vi "Bring UI To Front.vi"(11 "UI Data in":refnum<class "Settings UI.lvclass">) -> (0 "error out":errorcluster, 3 "UI Data out":refnum<class "Settings UI.lvclass">)   [LabVIEW 2020, in "Output Sequencer.lvlib" / "Settings UI.lvclass"]
uses:
  Settings UI.lvclass
  Settings UI.lvclass/Settings UI.ctl
  user32.dll
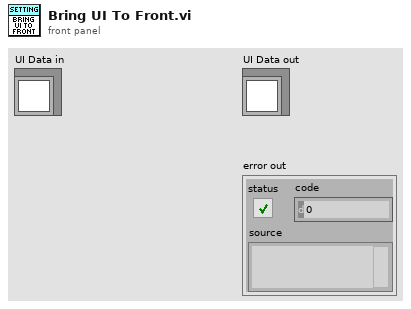
[diagram p1: front panel]
types:
  T1 = enum32{"Invalid", "Standard", "Closed", "Hidden", "Minimized", "Maximized"}
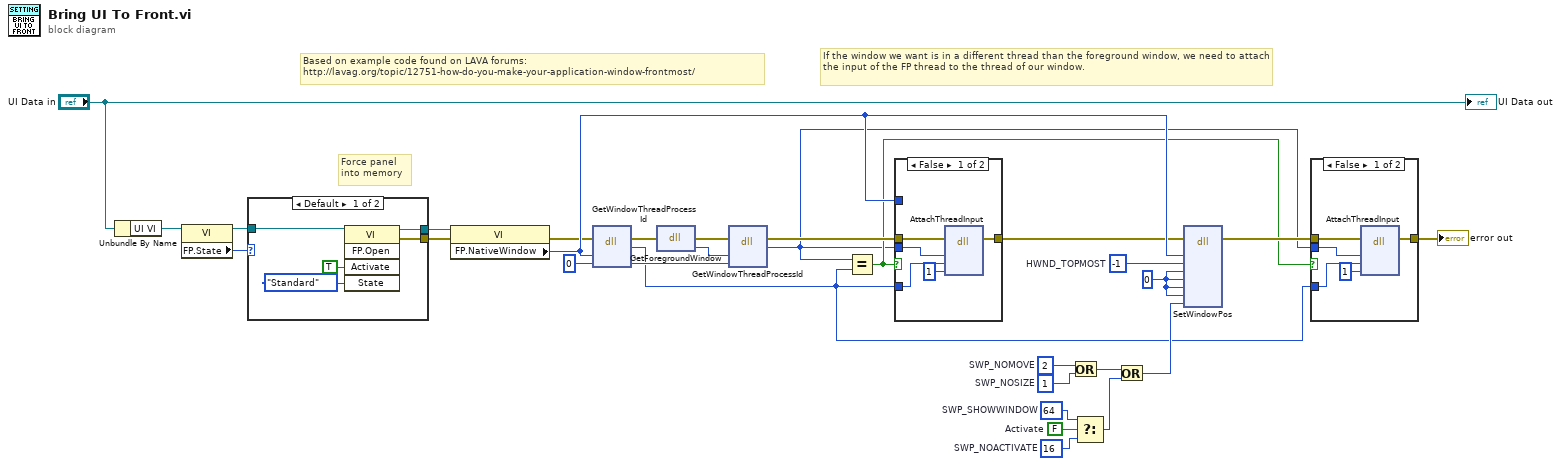
[diagram p0: block diagram]
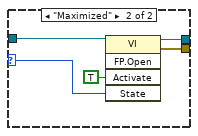
[diagram p2: hidden frame]
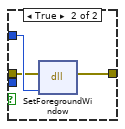
[diagram p4: hidden frame]
diagram:
  w14 = FALSE  # Activate
  w21 = -1  # HWND_TOPMOST
  w13 = u32 16  # SWP_NOACTIVATE
  w12 = u32 64  # SWP_SHOWWINDOW
  w18 = 0 ("lpdwProcessID")
  w26 = u32 2  # SWP_NOMOVE
  w25 = u32 1  # SWP_NOSIZE
  w27 = 0
  # "Force panel\ninto memory"
  # "Based on example code found on LAVA forums:\nhttp://lavag.org/topic/12751-how-do-you-make-your-application-window-frontmost/"
  # "If the window we want is in a different thread than the foreground window, we need to attach the input of the FP thread to the thread of our window."
  n1 = Unbundle By Name("UI Data in") -> ("UI VI"=w2:refnum<vi>)
  n2 = property class="VI"(reference=w2) -> (reference out=w7:refnum<vi>, "FP.State"=w6:T1)  [unwired: 1 in, 1 out]
  n3 = case shown="Default" w6 {
    selector: w6 -> [_ w35]
    tunnel: [w32 w38] -> w29
    tunnel: [w31 w37] -> w28
    tunnel: w7 -> [w30 w36]
    frame Default {
      n4 = invoke class="VI" method="FP.Open"(reference=w30, "Activate"=TRUE ("Activate?"), "State"=T1."Standard") -> (reference out=w31:refnum<vi>, error out=w32:errorcluster)  [unwired: 2 in, 3 out]
    }
    frame "Maximized" {
      n5 = invoke class="VI" method="FP.Open"(reference=w36, "Activate"=TRUE ("Activate?"), "State"=w35) -> (reference out=w37:refnum<vi>, error out=w38:errorcluster)  [unwired: 2 in, 3 out]
    }
  }
  n6 = property class="VI"(reference=w28, error in=w29) -> (error out=w4:errorcluster, "FP.NativeWindow"=w20:u64)  [unwired: 1 out]
  n7 = dll-call lib="user32" fn="GetWindowThreadProcessId" label="Get\nWindow\nThread\nProcess\nId"(error in=w4, "hWnd"=w20, "lpdwProcessID"=w18) -> (error out=w16:errorcluster, w9:i32)  [unwired: 4 in, 1 out]
  n8 = dll-call lib="user32" fn="GetForegroundWindow" label="Get\nForeground\nWindow"(error in=w16) -> (error out=w17:errorcluster, "hWnd"=w19:i32)  [unwired: 2 in, 1 out]
  n9 = dll-call lib="user32" fn="GetWindowThreadProcessId" label="Get\nWindow\nThread\nProcess\nId"(error in=w17, "hWnd"=w19, "lpdwProcessID"=w18) -> (error out=w15:errorcluster, w8:i32)  [unwired: 4 in, 1 out]
  n10 = Equal?(x=w8, y=w9) -> (x = y?=w10:bool)
  n11 = case shown="False" w10 {
    tunnel: w8 -> [w44 _]
    tunnel: w9 -> [w43 _]
    tunnel: w20 -> [_ w47]
    tunnel: w15 -> [w41 w46]
    tunnel: [w40 w45] -> w5
    frame False {
      n12 = dll-call lib="user32" fn="AttachThreadInput" label="Attach\nThread\nInput"(error in=w41, "idAttach"=w44, "idAttachTo"=w43, "fAttach"=1) -> (error out=w40:errorcluster)  [unwired: 6 in, 1 out]
    }
    frame True {
      n13 = dll-call lib="user32" fn="SetForegroundWindow" label="Set\nForeground\nWindow"(error in=w46, "hWnd"=w47) -> (error out=w45:errorcluster)  [unwired: 4 in, 1 out]
    }
  }
  n14 = Or(x=w26, y=w25) -> (x .or. y?=w23:u32)
  n15 = Select(t=w12, s=w14, f=w13) -> (s? t:f=w24:u32)
  n16 = Or(x=w23, y=w24) -> (x .or. y?=w22:u32)
  n17 = dll-call lib="USER32.DLL" fn="SetWindowPos"(error in=w5, "hWnd"=w20, "hWndInsertAfter"=w21, "left"=w27, "top"=w27, "width"=w27, "height"=w27, "fuFlags"=w22) -> (error out=w11:errorcluster)  [unwired: 8 in, 3 out]
  n18 = case shown="False" w10 {
    tunnel: w8 -> [w52 _]
    tunnel: w9 -> [w51 _]
    tunnel: w11 -> [w49 w53]
    tunnel: [w48 w53] -> w3
    frame False {
      n19 = dll-call lib="user32" fn="AttachThreadInput" label="Attach\nThread\nInput"(error in=w49, "idAttach"=w52, "idAttachTo"=w51, "fAttach"=1) -> (error out=w48:errorcluster)  [unwired: 6 in, 1 out]
    }
    frame True {
    }
  }
  "error out" <- w3
  "UI Data out" <- "UI Data in"
